vi "CreatePrivateEvents.vi"(8 "error in (no error)":errorcluster, 11 "MAUI":refnum<class "SMO.UI.MAUI.lvclass">) -> (0 "error out":errorcluster, 3 "MAUI out":refnum<class "SMO.UI.MAUI.lvclass">)   [LabVIEW 2019, in "SMO.UI.MAUI.lvclass"]
doc: "---------------------------------------------------------------\nJKI State Machine Objects™\nhttp://jki.net/state-machine-objects/\nCopyright (C) 2005-2015, JKI <info@jki.net>\nALL RIGHTS RESERVEDJKI State Machine Objects (SMO) 1.0.0.4\nJKI - JKI\nCopyright (c) 2015, JKI"
uses:
  SMO.UI.MAUI.lvclass
  Typedefs/PrivateEvents--SMO.UI.MAUI.SetEmbedded.ctl
  <userlib>/LevyLab/Embedded UI/SMO.UI.Embedded/SMO.UI.Embedded.lvclass
  Typedefs/PrivateEvents--SMO.UI.MAUI.GetEmbedded.ctl
  Typedefs/PrivateEvents--SMO.UI.MAUI.SetPanelData.ctl
  Typedefs/PanelData.ctl
  Typedefs/PrivateEvents--SMO.UI.MAUI.GetPanelData.ctl
  Typedefs/PrivateEvents--SMO.UI.MAUI.UpdatePanel.ctl
  Typedefs/PrivateEvents--SMO.UI.MAUI.OpenSubpanel.ctl
  Typedefs/PrivateEvents--SMO.UI.MAUI.GetDefaultSubpanel.ctl
  Typedefs/DefaultSubpanel.ctl
  Typedefs/PrivateEvents--SMO.UI.MAUI.SetDefaultSubpanel.ctl
  SMO.UI.MAUI.lvclass/SMO.UI.MAUI.ctl
  <vilib>/JKI/JKI SMO/SMO.UI/SMO.UI.lvclass
panel:
  # "For instructions on how to use the JKI State Machine Objects, examples and video tutorials, visit:\nhttp://jki.net/state-machine-objects/\n\nJKI State Machine Objects™\nhttp://jki.net/state-machine-objects/\nCopyright (C) 2005-2015, JKI <info@jki.net>\nALL RIGHTS RESERVED"
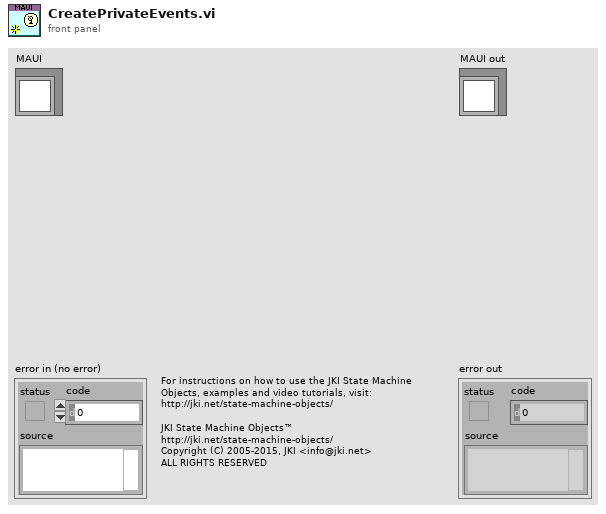
[diagram p1: front panel]
types:
  T1 = typedef "SMO.UI.MAUI.lvclass/PrivateEvents--SMO.UI.MAUI.SetDefaultSubpanel.ctl" = cluster{"Default Subpanel":cluster{"SMO.UI.Embedded":refnum<class "SMO.UI.Embedded.lvclass">}}
  T2 = typedef "SMO.UI.MAUI.lvclass/PrivateEvents--SMO.UI.MAUI.GetDefaultSubpanel.ctl" = refnum<notifier>
  T3 = typedef "SMO.UI.MAUI.lvclass/PrivateEvents--SMO.UI.MAUI.OpenSubpanel.ctl" = i32
  T4 = typedef "SMO.UI.MAUI.lvclass/PrivateEvents--SMO.UI.MAUI.UpdatePanel.ctl" = cluster{"Panel":i32, "Embedded":i32}
  T5 = typedef "SMO.UI.MAUI.lvclass/PrivateEvents--SMO.UI.MAUI.GetPanelData.ctl" = refnum<notifier>
  T6 = typedef "SMO.UI.MAUI.lvclass/PrivateEvents--SMO.UI.MAUI.SetPanelData.ctl" = T7[]
  T7 = typedef "SMO.UI.MAUI.lvclass/PanelData.ctl" = cluster{"SubPanel":refnum<vi>, "Ring":refnum<vi>, "Active":i32}
  T8 = typedef "SMO.UI.MAUI.lvclass/PrivateEvents--SMO.UI.MAUI.GetEmbedded.ctl" = cluster{"notifier out":refnum<notifier>}
  T9 = typedef "SMO.UI.MAUI.lvclass/PrivateEvents--SMO.UI.MAUI.SetEmbedded.ctl" = cluster{"Subpanels":refnum<class "SMO.UI.Embedded.lvclass">[]}
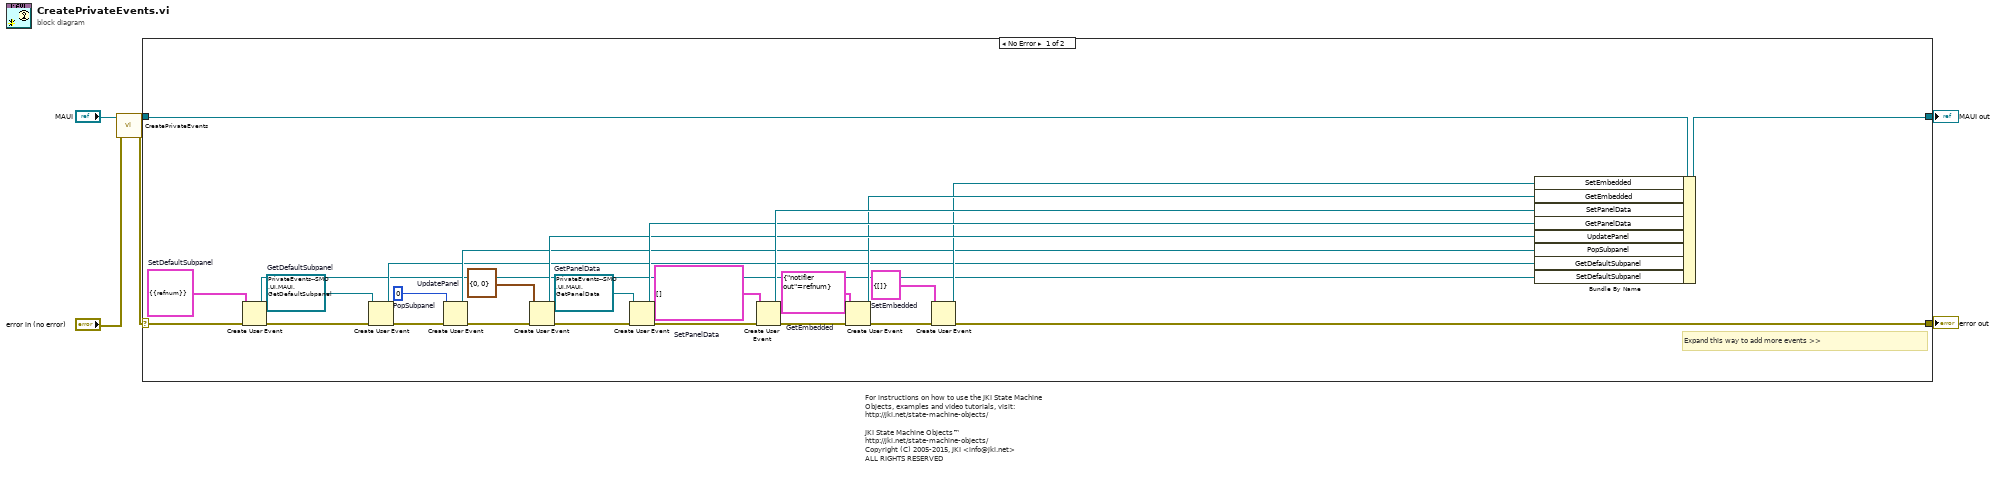
[diagram p0: block diagram]
diagram:
  # "For instructions on how to use the JKI State Machine Objects, examples and video tutorials, visit:\nhttp://jki.net/state-machine-objects/\n\nJKI State Machine Objects™\nhttp://jki.net/state-machine-objects/\nCopyright (C) 2005-2015, JKI <info@jki.net>\nALL RIGHTS RESERVED"
  n1 = call-parent "CreatePrivateEvents.vi"("error in (no error)"="error in (no error)", "SMO.UI"="MAUI") -> ("error out"=w1:errorcluster, "SMO.UI out"=w3:refnum<class "SMO.UI.MAUI.lvclass">)  [unwired: 8 in]
  n2 = case shown="No Error" w1 {
    selector: w1 -> [w32 w35]
    tunnel: [w19 w35] -> w5
    tunnel: [w31 w34] -> w6
    tunnel: w3 -> [w33 w34]
    frame No Error {
      w8 = T1 {"Default Subpanel"={"SMO.UI.Embedded"=refnum}}  # SetDefaultSubpanel
      w11 = T2 refnum  # GetDefaultSubpanel
      w14 = T3 0  # PopSubpanel
      w21 = T4 {"Panel"=0, "Embedded"=0}  # UpdatePanel
      w24 = T5 refnum  # GetPanelData
      w27 = T6 []  # SetPanelData
      w28 = T8 {"notifier out"=refnum}  # GetEmbedded
      w30 = T9 {"Subpanels"=[]}  # SetEmbedded
      # "Expand this way to add more events >>"
      n3 = Create User Event(user event datatype=w8, error in=w32) -> (user event=w7:refnum<user-event>, error out=w9:errorcluster)
      n4 = Create User Event(user event datatype=w11, error in=w9) -> (user event=w10:refnum<user-event>, error out=w12:errorcluster)
      n5 = Create User Event(user event datatype=w14, error in=w12) -> (user event=w13:refnum<user-event>, error out=w15:errorcluster)
      n6 = Create User Event(user event datatype=w21, error in=w15) -> (user event=w20:refnum<user-event>, error out=w22:errorcluster)
      n7 = Create User Event(user event datatype=w24, error in=w22) -> (user event=w23:refnum<user-event>, error out=w25:errorcluster)
      n8 = Create User Event(user event datatype=w27, error in=w25) -> (user event=w26:refnum<user-event>, error out=w18:errorcluster)
      n9 = Create User Event(user event datatype=w28, error in=w18) -> (user event=w17:refnum<user-event>, error out=w29:errorcluster)
      n10 = Create User Event(user event datatype=w30, error in=w29) -> (user event=w16:refnum<user-event>, error out=w19:errorcluster)
      n11 = Bundle By Name(cluster=w33, "SetEmbedded"=w16, "GetEmbedded"=w17, "SetPanelData"=w26, "GetPanelData"=w23, "UpdatePanel"=w20, "PopSubpanel"=w13, "GetDefaultSubpanel"=w10, "SetDefaultSubpanel"=w7) -> (w31:refnum<class "SMO.UI.MAUI.lvclass">)
    }
    frame Error {
    }
  }
  "error out" <- w5
  "MAUI out" <- w6
